vi "sendCenterTarget.vi"(11 "Target Info":T3(array[cluster])) -> (2 "Values":T2)   [LabVIEW 2012]
uses:
  typeDefs/targetVariables.ctl
panel:
  in  "Cluster 2":T1
  in  "Cluster":T2
  out "output variable":sgl
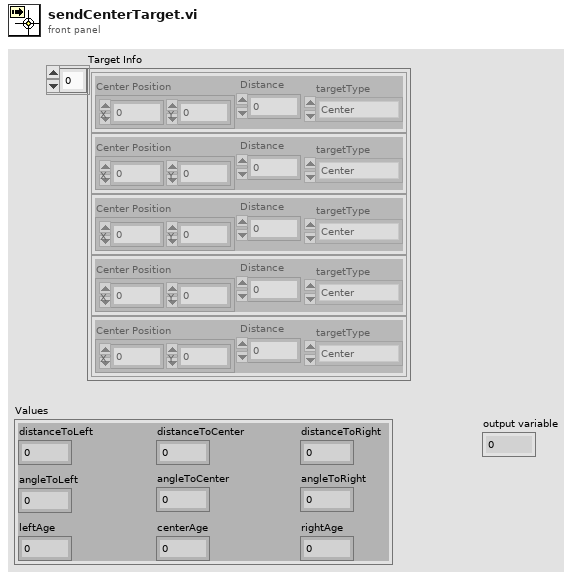
[diagram p1: front panel]
types:
  T1 = cluster{"centerRead":timestamp, "rightRead":timestamp, "leftRead":timestamp}
  T2 = typedef "targetVariables.ctl" = cluster{"distanceToCenter":dbl, "angleToCenter":dbl, "angleToLeft":dbl, "distanceToLeft":dbl, "angleToRight":dbl, "distanceToRight":dbl, "centerAge":dbl, "leftAge":dbl, "rightAge":dbl}
  T3 = cluster{"Center Position":cluster{"X":dbl, "Y":dbl}, "Distance":dbl, "targetType":enum16{"Center", "Side", "Vertical"}}[]
  T4 = enum16{"Invalid", "Center", "TwoSides", "TwoVerticals", "SideAndVert", "OneSide"}
  T5 = cluster{"Center Position":cluster{"X":dbl, "Y":dbl}, "Distance":dbl, "targetType":enum16{"Center", "Side", "Vertical"}}
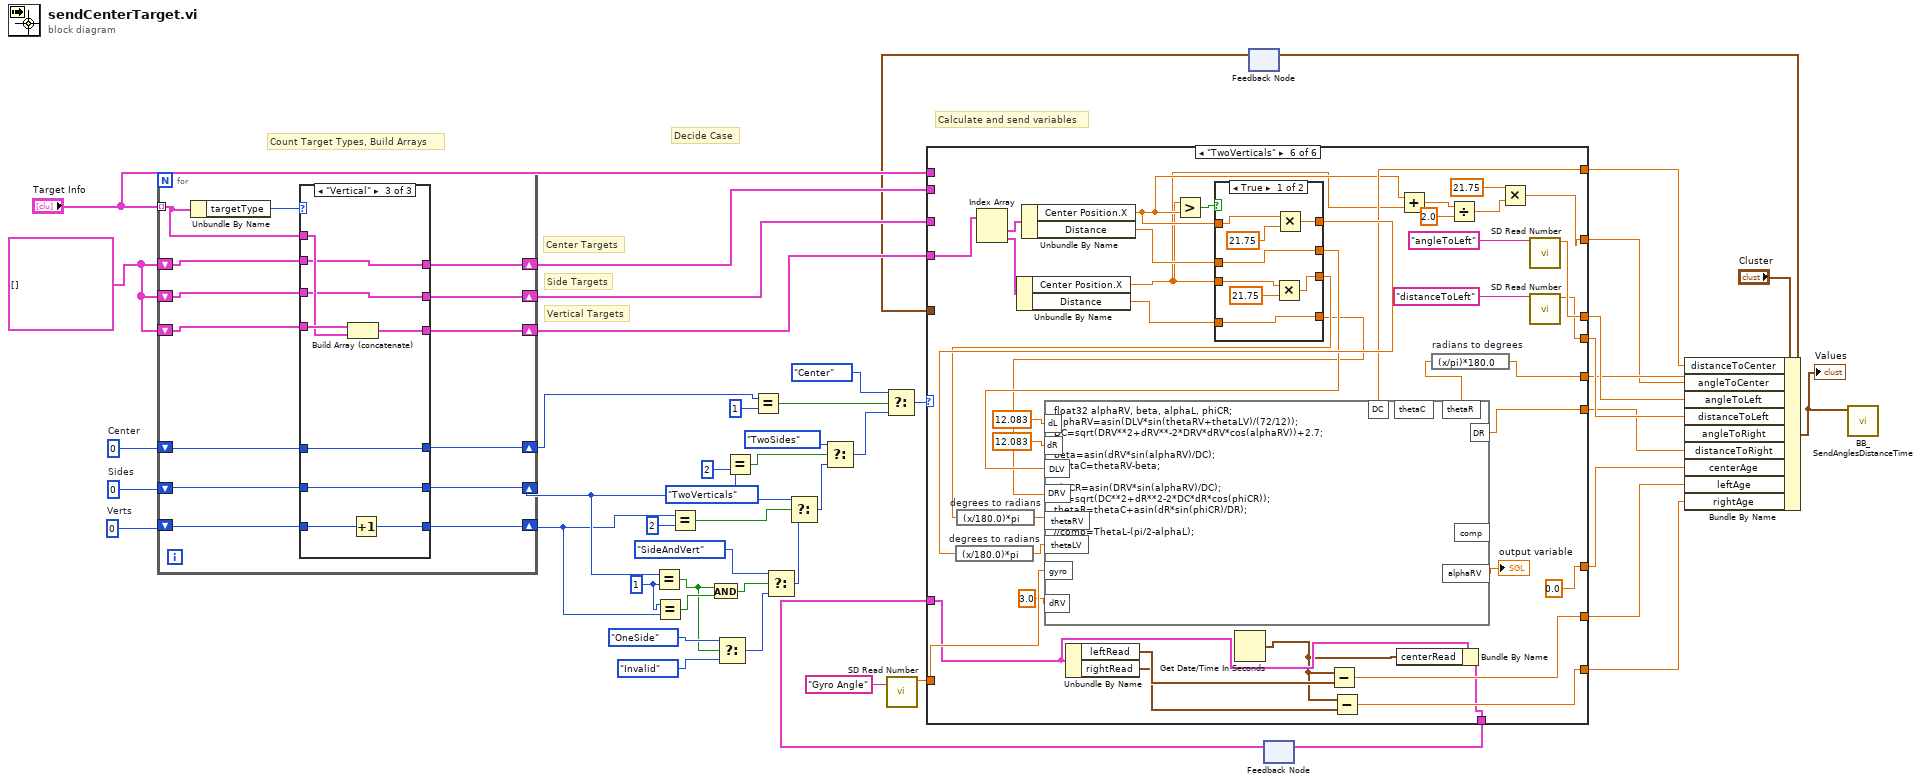
[diagram p0: block diagram]
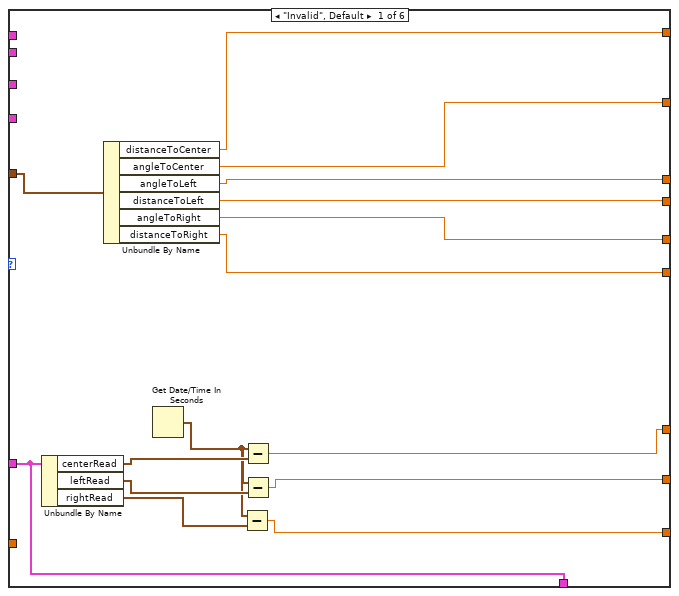
[diagram p2: hidden frame]
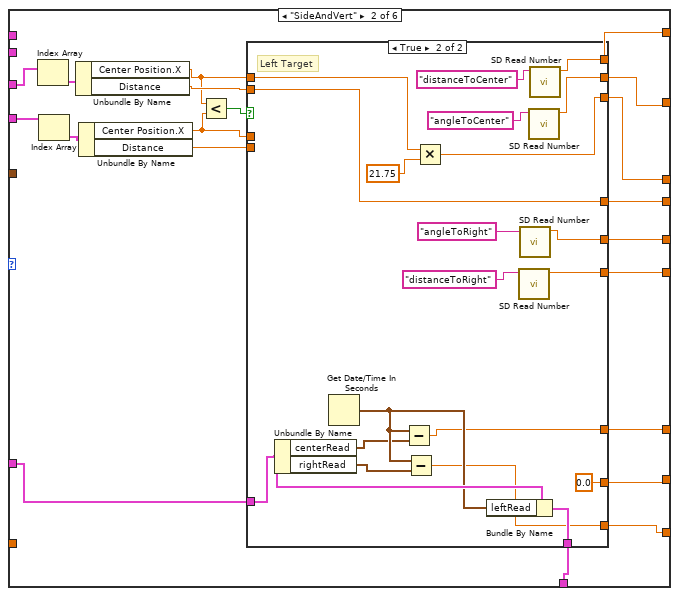
[diagram p3: hidden frame]
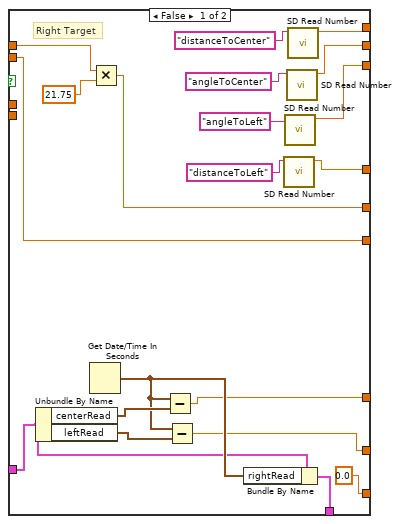
[diagram p4: hidden frame]
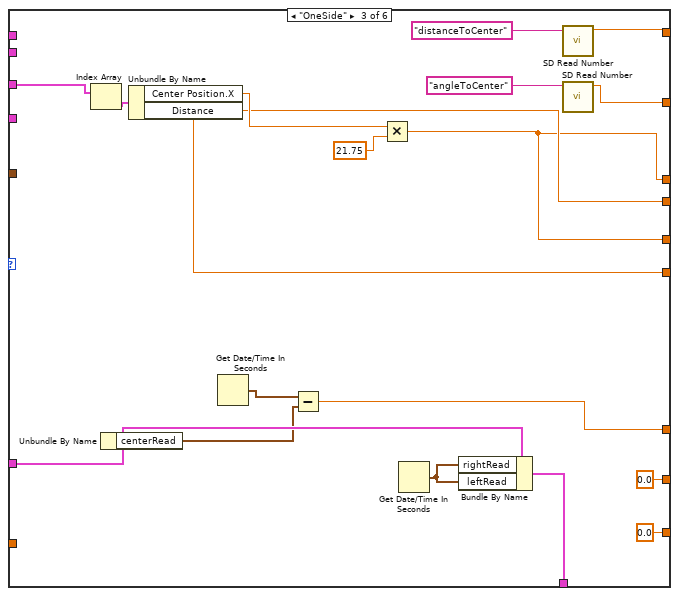
[diagram p5: hidden frame]
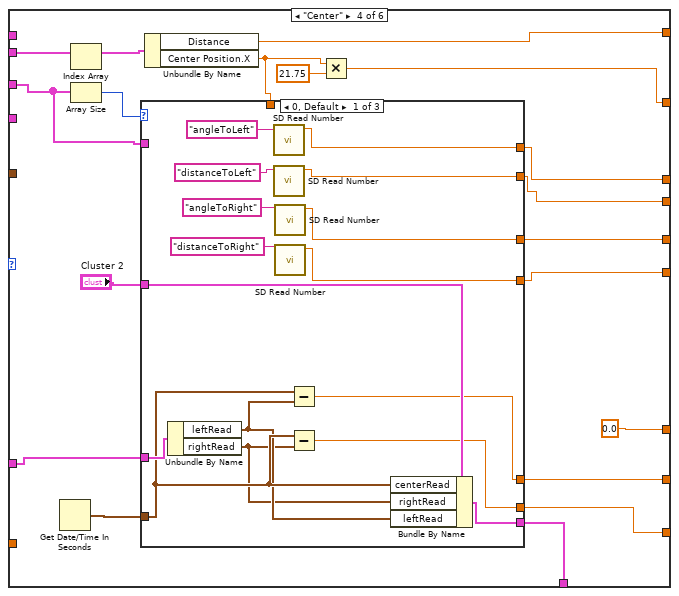
[diagram p6: hidden frame]
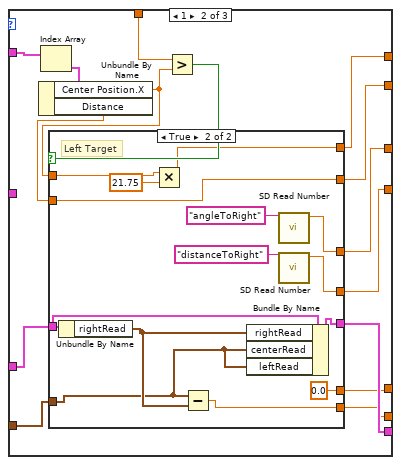
[diagram p7: hidden frame]
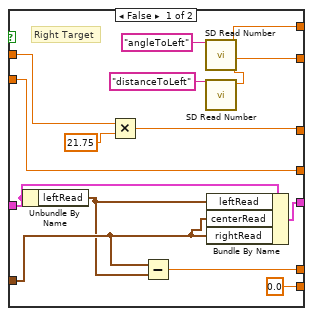
[diagram p8: hidden frame]
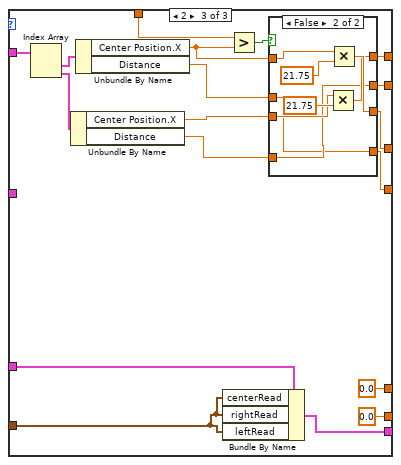
[diagram p9: hidden frame]
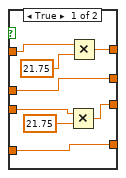
[diagram p10: hidden frame]
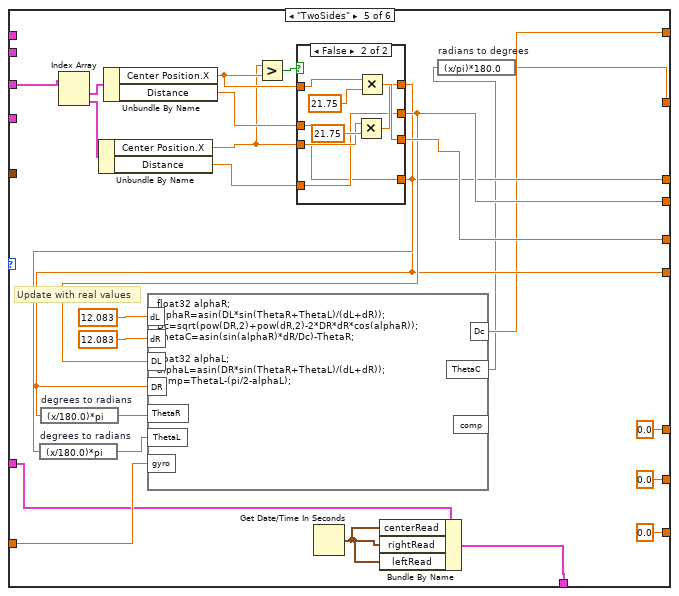
[diagram p11: hidden frame]
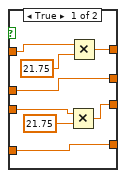
[diagram p12: hidden frame]
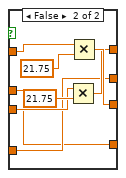
[diagram p13: hidden frame]
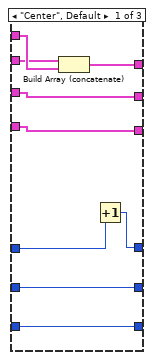
[diagram p14: hidden frame]
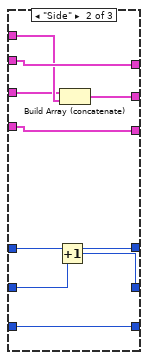
[diagram p15: hidden frame]
diagram:
  w20 = T3 []
  w28 = 1 ("y")
  w46 = 0  # Verts
  w47 = 0  # Sides
  w48 = 0  # Center
  # "Vertical Targets"
  # "Side Targets"
  # "Center Targets"
  # "Calculate and send variables"
  # "Decide Case"
  # "Count Target Types, Build Arrays"
  n1 = for {
    tunnel: "Target Info" -> [w55] mode=indexing
    shift-right: [w60] -> w38
    shift-left: w48 -> [w61]
    shift-right: [w59] -> w30
    shift-left: w47 -> [w58]
    shift-right: [w57] -> w29
    shift-left: w46 -> [w56]
    shift-right: [w54] -> w19
    shift-left: w20 -> [w53]
    shift-right: [w52] -> w18
    shift-left: w20 -> [w51]
    shift-right: [w50] -> w17
    shift-left: w20 -> [w49]
    n2 = Unbundle By Name(w55) -> ("targetType"=w62:enum16{"Center", "Side", "Vertical"})
    n3 = case shown="\"Vertical\"" w62 {
      tunnel: w61 -> [w71 w78 w87]
      tunnel: [w70 w78 w87] -> w60
      tunnel: [w69 w79 w86] -> w59
      tunnel: w58 -> [w69 w80 w86]
      tunnel: [w68 w77 w88] -> w57
      tunnel: w56 -> [w68 w77 w89]
      tunnel: w55 -> [w66 w75 w83]
      tunnel: [w67 w76 w82] -> w54
      tunnel: w53 -> [w65 w76 w82]
      tunnel: [w64 w74 w81] -> w52
      tunnel: w51 -> [w64 w73 w81]
      tunnel: [w63 w72 w85] -> w50
      tunnel: w49 -> [w63 w72 w84]
      frame "Center", Default {
        n4 = Build Array (concatenate)(w65, w66) -> (w67:T3)
        n5 = Increment(x=w71) -> (x+1=w70:i32)
      }
      frame "Side" {
        n6 = Increment(x=w80) -> (x+1=w79:i32)
        n7 = Build Array (concatenate)(w73, w75) -> (w74:T3)
      }
      frame "Vertical" {
        n8 = Build Array (concatenate)(w84, w83) -> (w85:T3)
        n9 = Increment(x=w89) -> (x+1=w88:i32)
      }
    }
  }
  n10 = Equal?(x=w30, y=w28) -> (x = y?=w23:bool)
  n11 = Equal?(x=w28, y=w29) -> (x = y?=w27:bool)
  n12 = Equal?(x=w29, y=2) -> (x = y?=w34:bool)
  n13 = And(x=w23, y=w27) -> (x .and. y?=w26:bool)
  n14 = Select(t=T4."OneSide" ("y"), s=w23, f=T4."Invalid" ("y")) -> (s? t:f=w25:T4)
  n15 = Equal?(x=w30, y=2) -> (x = y?=w36:bool)
  n16 = Equal?(x=w38, y=1) -> (x = y?=w39:bool)
  n17 = Select(t=T4."SideAndVert" ("y"), s=w26, f=w25) -> (s? t:f=w32:T4)
  n18 = Select(t=T4."TwoVerticals" ("y"), s=w34, f=w32) -> (s? t:f=w35:T4)
  n19 = Select(t=T4."TwoSides" ("y"), s=w36, f=w35) -> (s? t:f=w41:T4)
  n20 = Select(t=T4."Center" ("y"), s=w39, f=w41) -> (s? t:f=w43:T4)
  n21 = call <vilib>:"SD Read Number.vi"("Name"="Gyro Angle") -> ("Numeric"=w15:dbl)  [unwired: 8 in, 2 out]
  n22 = feedback #1() -> (w1:T2)  [unwired: 1 in]
  n23 = feedback #2() -> (w13:T1)  [unwired: 1 in]
  n24 = case shown="\"TwoVerticals\"" w43 {
    tunnel: "Target Info" -> [_ _ _ _ _ _]
    tunnel: [w94 w110 w175 w190 w303 w345] -> w3
    tunnel: w19 -> [_ _ _ w200 _ _]
    tunnel: w18 -> [_ w124 w165 w197 w320 _]
    tunnel: w17 -> [_ w123 _ _ _ w366]
    tunnel: [w91 w113 w179 w195 w319 w361] -> w9
    tunnel: [w93 w117 w179 w194 w306 w351] -> w11
    tunnel: [w95 w111 w176 w191 w304 w364] -> w12
    tunnel: [w90 w112 w180 w193 w305 w362] -> w8
    tunnel: [w92 w114 w180 w192 w311 w350] -> w10
    tunnel: w15 -> [_ _ _ _ w301 w367]
    tunnel: [w100 w106 w168 0.0 0.0 0.0] -> w7
    tunnel: [w97 w108 w172 w188 w296 w347] -> w14
    tunnel: w13 -> [w97 w109 w171 w185 w297 w348]
    tunnel: [w99 w107 0.0 w184 0.0 w355] -> w6
    tunnel: [w98 w105 0.0 ("y") w183 0.0 ("y") w354] -> w5
    tunnel: w1 -> [w96 _ _ _ _ _]
    frame "Invalid", Default {
      n25 = Unbundle By Name(w97) -> ("centerRead"=w104:timestamp, "leftRead"=w103:timestamp, "rightRead"=w101:timestamp)
      n26 = Unbundle By Name(w96) -> ("distanceToCenter"=w95:dbl, "angleToCenter"=w94:dbl, "angleToLeft"=w93:dbl, "distanceToLeft"=w92:dbl, "angleToRight"=w91:dbl, "distanceToRight"=w90:dbl)
      n27 = Get Date/Time In Seconds() -> (seconds since 1Jan1904=w102:timestamp)
      n28 = Subtract(x=w102, y=w101) -> (x-y=w98:dbl)
      n29 = Subtract(x=w102, y=w104) -> (x-y=w100:dbl)
      n30 = Subtract(x=w102, y=w103) -> (x-y=w99:dbl)
    }
    frame "SideAndVert" {
      n31 = Index Array(array=w124) -> (element=w122:T5)  [unwired: 1 in]
      n32 = Index Array(array=w123) -> (element=w121:T5)  [unwired: 1 in]
      n33 = Unbundle By Name(w122) -> ("Center Position.X"=w116:dbl, "Distance"=w119:dbl)
      n34 = Unbundle By Name(w121) -> ("Center Position.X"=w115:dbl, "Distance"=w118:dbl)
      n35 = Less?(x=w116, y=w115) -> (x < y?=w120:bool)
      n36 = case shown="True" w120 {
        tunnel: w116 -> [w143 w162]
        tunnel: w119 -> [w141 w161]
        tunnel: w115 -> [_ _]
        tunnel: w118 -> [_ _]
        tunnel: [w136 w163] -> w117
        tunnel: [w135 w161] -> w114
        tunnel: [w142 w158] -> w113
        tunnel: [w141 w157] -> w112
        tunnel: [w140 w154] -> w111
        tunnel: [w139 w153] -> w110
        tunnel: w109 -> [w128 w152]
        tunnel: [w129 w151] -> w108
        tunnel: [w126 0.0] -> w107
        tunnel: [w125 w146] -> w106
        tunnel: [0.0 w145] -> w105
        frame False {
          # "Right Target"
          n37 = Unbundle By Name(w128) -> ("centerRead"=w131:timestamp, "leftRead"=w132:timestamp)
          n38 = Get Date/Time In Seconds() -> (seconds since 1Jan1904=w130:timestamp)
          n39 = Multiply(x=w143, y=21.75) -> (x*y=w142:dbl)
          n40 = Subtract(x=w130, y=w131) -> (x-y=w125:dbl)
          n41 = Subtract(x=w130, y=w132) -> (x-y=w126:dbl)
          n42 = Bundle By Name(cluster=w128, "rightRead"=w130) -> (w129:T1)
          n43 = call <vilib>:"SD Read Number.vi"("Name"="distanceToLeft") -> ("Numeric"=w135:dbl)  [unwired: 8 in, 2 out]
          n44 = call <vilib>:"SD Read Number.vi"("Name"="angleToLeft") -> ("Numeric"=w136:dbl)  [unwired: 8 in, 2 out]
          n45 = call <vilib>:"SD Read Number.vi"("Name"="angleToCenter") -> ("Numeric"=w139:dbl)  [unwired: 8 in, 2 out]
          n46 = call <vilib>:"SD Read Number.vi"("Name"="distanceToCenter") -> ("Numeric"=w140:dbl)  [unwired: 8 in, 2 out]
        }
        frame True {
          # "Left Target"
          n47 = Unbundle By Name(w152) -> ("centerRead"=w148:timestamp, "rightRead"=w147:timestamp)
          n48 = Get Date/Time In Seconds() -> (seconds since 1Jan1904=w149:timestamp)
          n49 = Subtract(x=w149, y=w148) -> (x-y=w146:dbl)
          n50 = Subtract(x=w149, y=w147) -> (x-y=w145:dbl)
          n51 = Multiply(x=w162, y=21.75) -> (x*y=w163:dbl)
          n52 = Bundle By Name(cluster=w152, "leftRead"=w149) -> (w151:T1)
          n53 = call <vilib>:"SD Read Number.vi"("Name"="distanceToRight") -> ("Numeric"=w157:dbl)  [unwired: 8 in, 2 out]
          n54 = call <vilib>:"SD Read Number.vi"("Name"="angleToRight") -> ("Numeric"=w158:dbl)  [unwired: 8 in, 2 out]
          n55 = call <vilib>:"SD Read Number.vi"("Name"="angleToCenter") -> ("Numeric"=w153:dbl)  [unwired: 8 in, 2 out]
          n56 = call <vilib>:"SD Read Number.vi"("Name"="distanceToCenter") -> ("Numeric"=w154:dbl)  [unwired: 8 in, 2 out]
        }
      }
    }
    frame "OneSide" {
      n57 = Index Array(array=w165) -> (element=w166:T5)  [unwired: 1 in]
      n58 = Unbundle By Name(w171) -> ("centerRead"=w169:timestamp)
      n59 = Unbundle By Name(w166) -> ("Center Position.X"=w182:dbl, "Distance"=w180:dbl)
      n60 = Get Date/Time In Seconds() -> (seconds since 1Jan1904=w170:timestamp)
      n61 = Subtract(x=w170, y=w169) -> (x-y=w168:dbl)
      n62 = Multiply(x=w182, y=21.75) -> (x*y=w179:dbl)
      n63 = Get Date/Time In Seconds() -> (seconds since 1Jan1904=w167:timestamp)
      n64 = Bundle By Name(cluster=w171, "rightRead"=w167, "leftRead"=w167) -> (w172:T1)
      n65 = call <vilib>:"SD Read Number.vi"("Name"="distanceToCenter") -> ("Numeric"=w176:dbl)  [unwired: 8 in, 2 out]
      n66 = call <vilib>:"SD Read Number.vi"("Name"="angleToCenter") -> ("Numeric"=w175:dbl)  [unwired: 8 in, 2 out]
    }
    frame "Center" {
      n67 = Get Date/Time In Seconds() -> (seconds since 1Jan1904=w186:timestamp)
      n68 = Index Array(array=w200) -> (element=w199:T5)  [unwired: 1 in]
      n69 = Array Size(array=w197) -> (size(s)=w198:i32)
      n70 = Unbundle By Name(w199) -> ("Distance"=w191:dbl, "Center Position.X"=w196:dbl)
      n71 = case shown="0, Default" w198 {
        tunnel: w197 -> [_ w232 w278]
        tunnel: w196 -> [_ w230 w275]
        tunnel: [w209 w224 w272] -> w195
        tunnel: [w211 w227 w271] -> w194
        tunnel: [w208 w223 w269] -> w193
        tunnel: [w210 w228 w266] -> w192
        tunnel: [w217 w220 w264] -> w188
        tunnel: "Cluster 2" -> [w216 _ _]
        tunnel: w186 -> [w214 w221 w261]
        tunnel: w185 -> [w215 w222 w265]
        tunnel: [w213 w219 0.0] -> w184
        tunnel: [w212 w218 0.0 ("y")] -> w183
        frame 0, Default {
          n72 = Unbundle By Name(w215) -> ("leftRead"=w203:timestamp, "rightRead"=w202:timestamp)
          n73 = call <vilib>:"SD Read Number.vi"("Name"="angleToLeft") -> ("Numeric"=w211:dbl)  [unwired: 8 in, 2 out]
          n74 = call <vilib>:"SD Read Number.vi"("Name"="distanceToLeft") -> ("Numeric"=w210:dbl)  [unwired: 8 in, 2 out]
          n75 = call <vilib>:"SD Read Number.vi"("Name"="angleToRight") -> ("Numeric"=w209:dbl)  [unwired: 8 in, 2 out]
          n76 = call <vilib>:"SD Read Number.vi"("Name"="distanceToRight") -> ("Numeric"=w208:dbl)  [unwired: 8 in, 2 out]
          n77 = Subtract(x=w214, y=w203) -> (x-y=w213:dbl)
          n78 = Subtract(x=w214, y=w202) -> (x-y=w212:dbl)
          n79 = Bundle By Name(cluster=w216, "centerRead"=w214, "rightRead"=w202, "leftRead"=w203) -> (w217:T1)
        }
        frame 1 {
          n80 = Index Array(array=w232) -> (element=w231:T5)  [unwired: 1 in]
          n81 = Unbundle By Name(w231) -> ("Center Position.X"=w225:dbl, "Distance"=w226:dbl)
          n82 = Greater?(x=w230, y=w225) -> (0:w229:bool)
          n83 = case shown="True" w229 {
            tunnel: [w239 w260] -> w228
            tunnel: w226 -> [w246 w260]
            tunnel: w225 -> [w243 w258]
            tunnel: [w240 w257] -> w227
            tunnel: [w244 w254] -> w224
            tunnel: [w246 w253] -> w223
            tunnel: w222 -> [w238 w252]
            tunnel: w221 -> [w236 w248]
            tunnel: [w237 w251] -> w220
            tunnel: [w234 0.0] -> w219
            tunnel: [0.0 ("y") w249] -> w218
            frame False {
              # "Right Target"
              n84 = Unbundle By Name(w238) -> ("leftRead"=w235:timestamp)
              n85 = Multiply(x=w243, y=21.75) -> (x*y=w244:dbl)
              n86 = Subtract(x=w236, y=w235) -> (x-y=w234:dbl)
              n87 = call <vilib>:"SD Read Number.vi"("Name"="angleToLeft") -> ("Numeric"=w240:dbl)  [unwired: 8 in, 2 out]
              n88 = call <vilib>:"SD Read Number.vi"("Name"="distanceToLeft") -> ("Numeric"=w239:dbl)  [unwired: 8 in, 2 out]
              n89 = Bundle By Name(cluster=w238, "leftRead"=w235, "centerRead"=w236, "rightRead"=w236) -> (w237:T1)
            }
            frame True {
              # "Left Target"
              n90 = Unbundle By Name(w252) -> ("rightRead"=w250:timestamp)
              n91 = Multiply(x=w258, y=21.75) -> (x*y=w257:dbl)
              n92 = Subtract(x=w248, y=w250) -> (x-y=w249:dbl)
              n93 = Bundle By Name(cluster=w252, "rightRead"=w250, "centerRead"=w248, "leftRead"=w248) -> (w251:T1)
              n94 = call <vilib>:"SD Read Number.vi"("Name"="angleToRight") -> ("Numeric"=w254:dbl)  [unwired: 8 in, 2 out]
              n95 = call <vilib>:"SD Read Number.vi"("Name"="distanceToRight") -> ("Numeric"=w253:dbl)  [unwired: 8 in, 2 out]
            }
          }
        }
        frame 2 {
          n96 = Index Array(array=w278) -> (element #1=w277:T5, element #2=w276:T5)  [unwired: 2 in]
          n97 = Unbundle By Name(w276) -> ("Center Position.X"=w273:dbl, "Distance"=w268:dbl)
          n98 = Unbundle By Name(w277) -> ("Center Position.X"=w270:dbl, "Distance"=w267:dbl)
          n99 = Bundle By Name(cluster=w265, "centerRead"=w261, "rightRead"=w261, "leftRead"=w261) -> (w264:T1)
          n100 = Greater?(x=w275, y=w270) -> (0:w274:bool)
          n101 = case shown="False" w274 {
            tunnel: w273 -> [w284 w292]
            tunnel: [w283 w290] -> w272
            tunnel: [w282 w289] -> w271
            tunnel: w270 -> [w281 w291]
            tunnel: [w280 w287] -> w269
            tunnel: w268 -> [w280 w288]
            tunnel: w267 -> [w279 w287]
            tunnel: [w279 w288] -> w266
            frame True {
              n102 = Multiply(x=w284, y=21.75) -> (x*y=w283:dbl)
              n103 = Multiply(x=w281, y=21.75) -> (x*y=w282:dbl)
            }
            frame False {
              n104 = Multiply(x=w292, y=21.75) -> (x*y=w289:dbl)
              n105 = Multiply(x=w291, y=21.75) -> (x*y=w290:dbl)
            }
          }
        }
      }
      n106 = Multiply(x=w196, y=21.75) -> (x*y=w190:dbl)
    }
    frame "TwoSides" {
      # "Update with real values"
      n107 = Index Array(array=w320) -> (element #1=w318:T5, element #2=w317:T5)  [unwired: 2 in]
      n108 = Unbundle By Name(w317) -> ("Center Position.X"=w312:dbl, "Distance"=w314:dbl)
      n109 = Unbundle By Name(w318) -> ("Center Position.X"=w315:dbl, "Distance"=w313:dbl)
      n110 = Greater?(x=w312, y=w315) -> (0:w316:bool)
      n111 = case shown="False" w316 {
        tunnel: w312 -> [w326 w334]
        tunnel: [w325 w332] -> w319
        tunnel: [w324 w331] -> w306
        tunnel: w315 -> [w323 w333]
        tunnel: [w322 w329] -> w305
        tunnel: w314 -> [w322 w330]
        tunnel: w313 -> [w321 w329]
        tunnel: [w321 w330] -> w311
        frame True {
          n112 = Multiply(x=w326, y=21.75) -> (x*y=w325:dbl)
          n113 = Multiply(x=w323, y=21.75) -> (x*y=w324:dbl)
        }
        frame False {
          n114 = Multiply(x=w334, y=21.75) -> (x*y=w331:dbl)
          n115 = Multiply(x=w333, y=21.75) -> (x*y=w332:dbl)
        }
      }
      n116 = expression code="(x/180.0)*pi" "degrees to radians"(w306) -> (w307:dbl)
      n117 = expression code="(x/180.0)*pi" "degrees to radians"(w305) -> (w308:dbl)
      n118 = formula code="float32 alphaR;\nalphaR=asin(DL*sin(ThetaR+ThetaL)/(dL+dR));\nDc=sqrt(pow(DR,2)+pow(dR,2)-2*DR*dR*cos(alphaR));\nThetaC=asin(sin(alphaR)*dR/Dc)-ThetaR;\n\nfloat32 alphaL;\nalphaL=asin(DR*sin(ThetaR+ThetaL)/(dL+dR));\ncomp=ThetaL-(pi/2-alphaL);"("dL"=12.083 ("input variable"), "dR"=12.083 ("input variable"), "DL"=w311, "DR"=w305, "ThetaR"=w308, "ThetaL"=w307, "gyro"=w301) -> ("Dc"=w304:dbl, "ThetaC"=w302:dbl)  [unwired: 1 out]
      n119 = Get Date/Time In Seconds() -> (seconds since 1Jan1904=w295:timestamp)
      n120 = Bundle By Name(cluster=w297, "centerRead"=w295, "rightRead"=w295, "leftRead"=w295) -> (w296:T1)
      n121 = expression code="(x/pi)*180.0" "radians to degrees"(w302) -> (w303:dbl)
    }
    frame "TwoVerticals" {
      n122 = Index Array(array=w366) -> (element #1=w376:T5, element #2=w375:T5)  [unwired: 2 in]
      n123 = Unbundle By Name(w375) -> ("Center Position.X"=w337:dbl, "Distance"=w373:dbl)
      n124 = Unbundle By Name(w376) -> ("Center Position.X"=w338:dbl, "Distance"=w372:dbl)
      n125 = Unbundle By Name(w348) -> ("leftRead"=w357:timestamp, "rightRead"=w356:timestamp)
      n126 = Greater?(x=w337, y=w338) -> (0:w374:bool)
      n127 = case shown="True" w374 {
        tunnel: w337 -> [w382 w390]
        tunnel: [w381 w388] -> w359
        tunnel: [w380 w387] -> w365
        tunnel: w338 -> [w379 w389]
        tunnel: [w378 w385] -> w339
        tunnel: w373 -> [w378 w386]
        tunnel: w372 -> [w377 w385]
        tunnel: [w377 w386] -> w340
        frame True {
          n128 = Multiply(x=w382, y=21.75) -> (x*y=w381:dbl)
          n129 = Multiply(x=w379, y=21.75) -> (x*y=w380:dbl)
        }
        frame False {
          n130 = Multiply(x=w390, y=21.75) -> (x*y=w387:dbl)
          n131 = Multiply(x=w389, y=21.75) -> (x*y=w388:dbl)
        }
      }
      n132 = expression code="(x/180.0)*pi" "degrees to radians"(w365) -> (w368:dbl)
      n133 = expression code="(x/180.0)*pi" "degrees to radians"(w359) -> (w369:dbl)
      n134 = formula code="float32 alphaRV, beta, alphaL, phiCR;\nalphaRV=asin(DLV*sin(thetaRV+thetaLV)/(72/12));\nDC=sqrt(DRV**2+dRV**-2*DRV*dRV*cos(alphaRV))+2.7;\n\nbeta=asin(dRV*sin(alphaRV)/DC);\nthetaC=thetaRV-beta;\n\nphiCR=asin(DRV*sin(alphaRV)/DC);\nDR=sqrt(DC**2+dR**2-2*DC*dR*cos(phiCR));\nthetaR=thetaC+asin(dR*sin(phiCR)/DR);\n\n//comp=ThetaL-(pi/2-alphaL);"("dL"=12.083 ("input variable"), "dR"=12.083 ("input variable"), "DLV"=w340, "DRV"=w339, "thetaRV"=w369, "thetaLV"=w368, "gyro"=w367, "dRV"=3.0 ("input variable")) -> ("DC"=w364:dbl, "DR"=w362:dbl, "thetaR"=w360:dbl, "alphaRV"=→"output variable":sgl)  [unwired: 2 out]
      n135 = Get Date/Time In Seconds() -> (seconds since 1Jan1904=w346:timestamp)
      n136 = Subtract(x=w346, y=w357) -> (x-y=w355:dbl)
      n137 = Subtract(x=w346, y=w356) -> (x-y=w354:dbl)
      n138 = Bundle By Name(cluster=w348, "centerRead"=w346) -> (w347:T1)
      n139 = Add(x=w338, y=w337) -> (x+y=w342:dbl)
      n140 = expression code="(x/pi)*180.0" "radians to degrees"(w360) -> (w361:dbl)
      n141 = Divide(x=w342, y=2.0) -> (x/y=w343:dbl)
      n142 = Multiply(x=21.75 ("y"), y=w343) -> (x*y=w345:dbl)
      n143 = call <vilib>:"SD Read Number.vi"("Name"="angleToLeft") -> ("Numeric"=w351:dbl)  [unwired: 8 in, 2 out]
      n144 = call <vilib>:"SD Read Number.vi"("Name"="distanceToLeft") -> ("Numeric"=w350:dbl)  [unwired: 8 in, 2 out]
    }
  }
  n145 = feedback-in #2(w14) -> ()
  n146 = Bundle By Name(cluster="Cluster", "distanceToCenter"=w12, "angleToCenter"=w3, "angleToLeft"=w11, "distanceToLeft"=w10, "angleToRight"=w9, "distanceToRight"=w8, "centerAge"=w7, "leftAge"=w6, "rightAge"=w5) -> (w2:T2)
  "Values" <- w2
  n147 = feedback-in #1(w2) -> ()
  n148 = call "BB_SendAnglesDistanceTime.vi"("Cluster"=w2) -> ()  [unwired: 11 in]
